vi "Match Values to Params.vi"(8 "error in (no error)":errorcluster, 10 "APU Sensor Info":string[][](array[string]), 11 "Cluster of Value Arrays":variant) -> (0 "error out":errorcluster, 3 "Params with Vals":T1[](array[typedef]))   [LabVIEW 2018, in "RT - Analysis.lvlib"]
doc: "Uses the APU Setup info to match parameters (Indicator Name) with their tags. It outputs all parameters with their value as a 1D array."
uses:
  RT - Analysis.lvlib
  Private Controls/Param Val Cluster.ctl
  Top Level/Shared VIs/Val Change Checker.vi
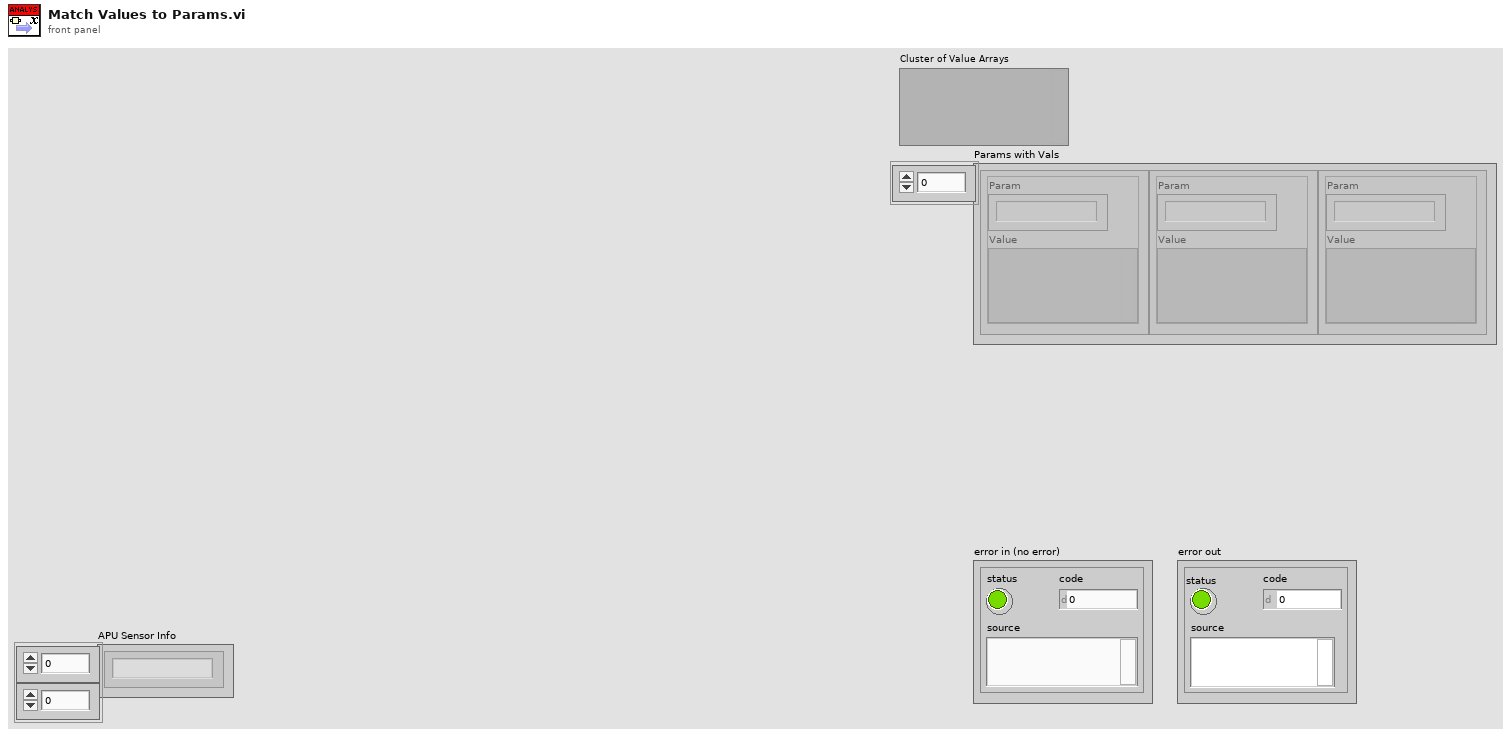
[diagram p1: front panel]
types:
  T1 = typedef "RT - Analysis.lvlib/Param Val Cluster.ctl" = cluster{"Param":string, "Value":variant}
  T2 = typedef "Parsed Tag Cluster.ctl" = cluster{"Whole Tag":string, "# of Sections":u8, "Chassis":u8, "Slot":u8, "Module":string, "Channel":u8, "SubChannel":u8}
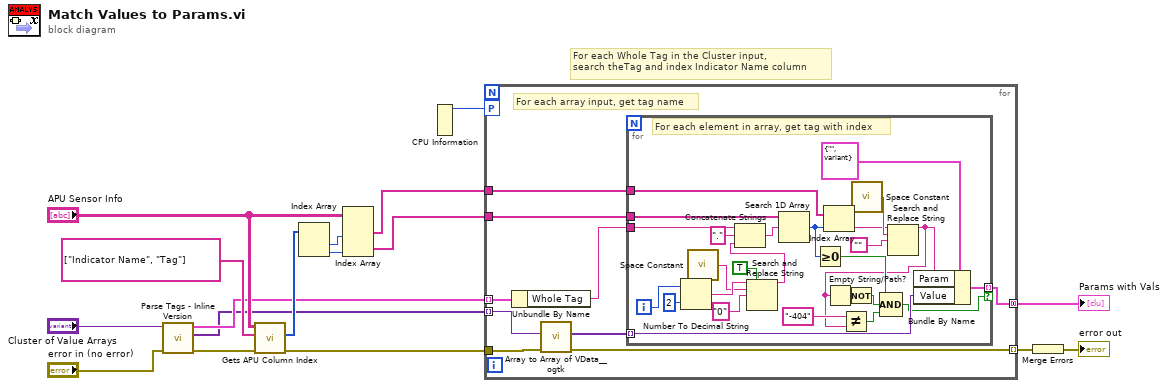
[diagram p0: block diagram]
diagram:
  # "For each Whole Tag in the Cluster input,\nsearch theTag and index Indicator Name column"
  n1 = call "Parse Tags - Inline Version.vi"("error in (no error)"="error in (no error)", "Cluster of Controls"="Cluster of Value Arrays") -> ("error out"=w14:errorcluster, "[VData out]"=w2:variant[], "[Parsed Tags]"=w3:T2[])  [unwired: 6 in, 1 out]
  n2 = call "Gets APU Column Index.vi"("error in (no error)"=w14, "[Column Names]"=string[] ["Indicator Name", "Tag"], "[[Array of Info]]"="APU Sensor Info") -> ("error out"=w4:errorcluster, "[Col Indices]"=w11:i32[])  [unwired: 4 in, 3 out]
  n3 = Index Array(array=w11) -> (element #1=w10:i32, element #2=w9:i32)  [unwired: 2 in]
  n4 = Index Array(array="APU Sensor Info", index (col) #1=w10, index (col) #2=w9) -> (element #1=w7:string[], element #2=w8:string[])  [unwired: 2 in]
  n5 = CPU Information() -> (4:w1:i32)  [unwired: 3 out]
  n6 = for {
    tunnel: w3 -> [w26] mode=indexing
    tunnel: w2 -> [w21] mode=indexing
    tunnel: w7 -> [w23]
    tunnel: w8 -> [w25]
    tunnel: [w22] -> w16 mode=concatenating
    tunnel: w4 -> [w20]
    tunnel: [w19] -> w6 mode=indexing
    workers-P: w1 -> [_]
    # "For each array input, get tag name"
    n7 = Unbundle By Name(w26) -> ("Whole Tag"=w24:string)
    n8 = call <userlib>:"Array to Array of VData__ogtk.vi"("error in (no error)"=w20, "MultiD Array"=w21) -> ("error out"=w19:errorcluster, "1D Array of Variants"=w18:variant[])  [unwired: 8 in]
    n9 = for {
      tunnel: w25 -> [w52]
      tunnel: w24 -> [w43]
      tunnel: w23 -> [w51]
      tunnel: [w49] -> w22 mode=indexing if=w33
      tunnel: w18 -> [w37] mode=indexing
      i -> [w48]
      # "For each element in array, get tag with index"
      n10 = Number To Decimal String(number=w48, width (-)=i16 2) -> (decimal integer string=w46:string)
      n11 = call <vilib>:"Space Constant.vi"() -> ("String"=w45:string)
      n12 = Search and Replace String(replace all?=TRUE ("replace all? (F)"), input string=w46, search string=w45, replace string="0" ("replace string (\"\")")) -> (result string=w42:string)  [unwired: 4 in, 3 out]
      n13 = Concatenate Strings(w43, "." ("string"), w42) -> (w39:string)
      n14 = Search 1D Array(1D array=w52, element=w39) -> (index of element=w38:i32)  [unwired: 1 in]
      n15 = Greater Or Equal To 0?(x=w38) -> (x >= 0?=w32:bool)
      n16 = Index Array(array=w51, index=w38) -> (element=w28:string)
      n17 = call <vilib>:"Space Constant.vi"() -> ("String"=w30:string)
      n18 = Search and Replace String(input string=w28, search string=w30, replace string="") -> (result string=w27:string)  [unwired: 5 in, 3 out]
      n19 = Empty String/Path?(string/path=w27) -> (empty?=w35:bool)
      n20 = Not Equal?(x="-404", y=w27) -> (x != y?=w36:bool)
      n21 = Not(x=w35) -> (.not. x?=w31:bool)
      n22 = Compound Arithmetic op=AND(w32, w31, w36) -> (w33:bool)
      n23 = Bundle By Name(cluster=T1 {"Param"="", "Value"=variant}, "Param"=w27, "Value"=w37) -> (w49:T1)
    }
  }
  "Params with Vals" <- w16
  n24 = Merge Errors(w6) -> (→"error out":errorcluster)
